vi "LV86_Combine Planes.vi"(2 "Blue":T1 {"Dialogs" format="%.0b"}, 3 "Green":T1 {"Dialogs" format="%.0b"}, 4 "Red":T1 {"Dialogs" format="%.0b"}) -> (1 "Image 2":T1 {"Dialogs" format="%.0b"})   [LabVIEW 2024]
doc: "This VI combines 3 greyscale images to make a color image"
uses:
  <userlib>/ImageProcessing/QTLIB_2595_LV86/QT_Image.ctl
panel:
  # "This VI combines 3 greyscale images to make a color image"
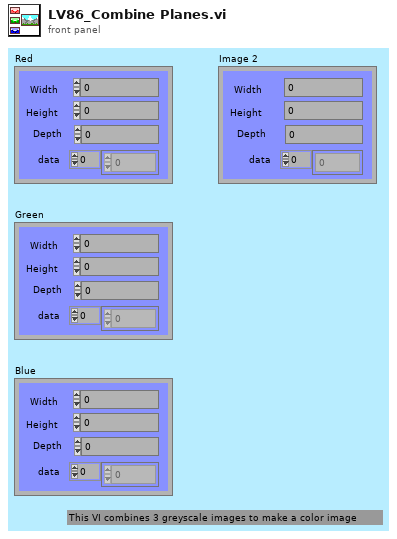
[diagram p1: front panel]
types:
  T1 = typedef "QT_Image.ctl" = cluster{"Width":i32, "Height":i32, "Depth":i32, "data":u8[], "Compressed data":u8[], "Color table":u32[], "Duration":i32, "Options":i32, "Timestamp":i32, "ID":i32, "Reserved":i32, "Dialogs":u32}
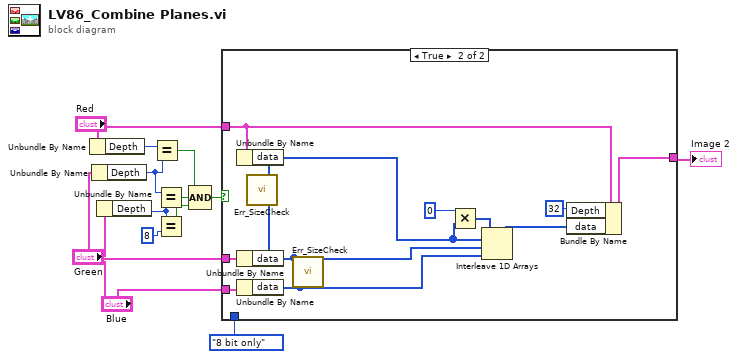
[diagram p0: block diagram]
diagram:
  n1 = Unbundle By Name("Red") -> ("Depth"=w7:i32)
  n2 = Unbundle By Name("Green") -> ("Depth"=w6:i32)
  n3 = Unbundle By Name("Blue") -> ("Depth"=w5:i32)
  n4 = Equal?(x=w7, y=w6) -> (x = y?=w3:bool)
  n5 = Equal?(x=w6, y=w5) -> (x = y?=w2:bool)
  n6 = Equal?(x=w5, y=u32 8) -> (x = y?=w1:bool)
  n7 = Compound Arithmetic op=AND(w3, w2, w1) -> (w12:bool)
  n8 = case shown="True" w12 {
    tunnel: [w14 w25] -> w13
    tunnel: "Red" -> [w14 w24]
    tunnel: "Green" -> [_ w23]
    tunnel: "Blue" -> [_ w22]
    tunnel: enum16{"Same depth", "8 bit only"}."8 bit only" ("Task") -> [_ _]
    frame False {
    }
    frame True {
      n9 = Unbundle By Name(w24) -> ("data"=w21:u8[])
      n10 = Unbundle By Name(w23) -> ("data"=w15:u8[])
      n11 = Unbundle By Name(w22) -> ("data"=w16:u8[])
      n12 = call <userlib>:"Err_SizeCheck.vi"("data 2"=w15, "data"=w21) -> ()  [unwired: 2 out]
      n13 = call <userlib>:"Err_SizeCheck.vi"("data 2"=w16, "data"=w15) -> ()  [unwired: 2 out]
      n14 = Multiply(x=u32 0, y=w21) -> (x*y=w17:u32[])
      n15 = Interleave 1D Arrays(w17, w21, w15, w16) -> (w20:u32[])
      n16 = Bundle By Name(cluster=w24, "Depth"=u32 32, "data"=w20) -> (w25:T1)
    }
  }
  "Image 2" <- w13
